vi "Instrument.Lockin.TestLauncher.vi"() -> ()   [LabVIEW 2019, in "Instrument.Lockin.lvlib" / "Instrument.Lockin.lvclass"]
uses:
  Instrument.Lockin.lvclass
  Instrument UI.Lockin/Instrument UI.Lockin.lvclass
  <userlib>/LevyLab/Instrument Framework/Instrument UI/Instrument UI.lvclass
  <userlib>/LevyLab/Instrument Framework/Instrument/Instrument.lvclass
  C:/Program Files (x86)/National Instruments/LabVIEW 2019/user.lib/LevyLab/Instrument Framework/Instrument Types/Lockin/Instrument.LockinAPI.lvclass
  C:/Program Files (x86)/National Instruments/LabVIEW 2019/user.lib/LevyLab/Instrument Framework/Instrument/Instrument.lvclass
  C:/Program Files (x86)/National Instruments/LabVIEW 2019/vi.lib/JKI/JKI SMO/SMO/SMO.lvclass
  <vilib>/JKI/JKI SMO/SMO/SMO.lvclass
  <vilib>/JKI/JKI SMO/SMO.UI/SMO.UI.lvclass
  <vilib>/JKI/JKI SMO/SMO/Typedefs/SMOState --Enum.ctl
  C:/Program Files (x86)/National Instruments/LabVIEW 2019/user.lib/LevyLab/Instrument Framework/Instrument UI/Instrument UI.lvclass
  C:/Program Files (x86)/National Instruments/LabVIEW 2019/vi.lib/JKI/JKI SMO/SMO.UI/SMO.UI.lvclass
  <vilib>/JKI/JKI SMO/SMO/Typedefs/Reserve State--Enum.ctl
  <vilib>/JKI/JKI SMO/SMO/Typedefs/Public Events.ctl
panel:
  out "String":string
  in  "Debug Mode? [F]":bool
  out "UI SMO State":T1
  out "SMO State":T1
  out "error out":errorcluster
  in  "Stop":bool
  # "Example Instrument SMO Test Launcher"
  # "For instructions on how to use the JKI State Machine Objects, examples and video tutorials, visit:\nhttp://jki.net/state-machine-objects/\n\nJKI State Machine Objects™\nhttp://jki.net/state-machine-objects/\nCopyright (C) 2005-2015, JKI <info@jki.net>\nALL RIGHTS RESERVED"
  # "Starting Example Instrument..."
  # "Close Panel to stop the SMO\n(press the \"X\")"
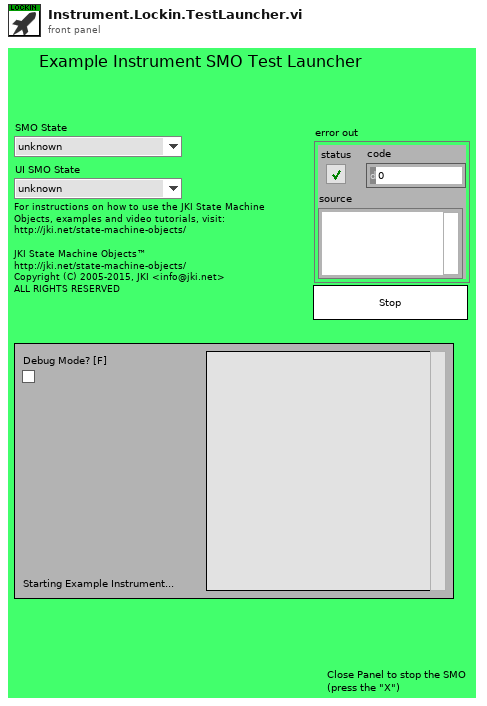
[diagram p1: front panel]
types:
  T1 = typedef "SMO.lvclass/SMOState --Enum.ctl" = enum16{"unknown", "Created", "Started", "Stopped"}
  T2 = typedef "SMO.lvclass/Public Events.ctl" = cluster{"Error":refnum<user-event>, "State":refnum<user-event>, "Reserve State":refnum<user-event>}
  T3 = enum32{"Invalid", "Standard", "Closed", "Hidden", "Minimized", "Maximized"}
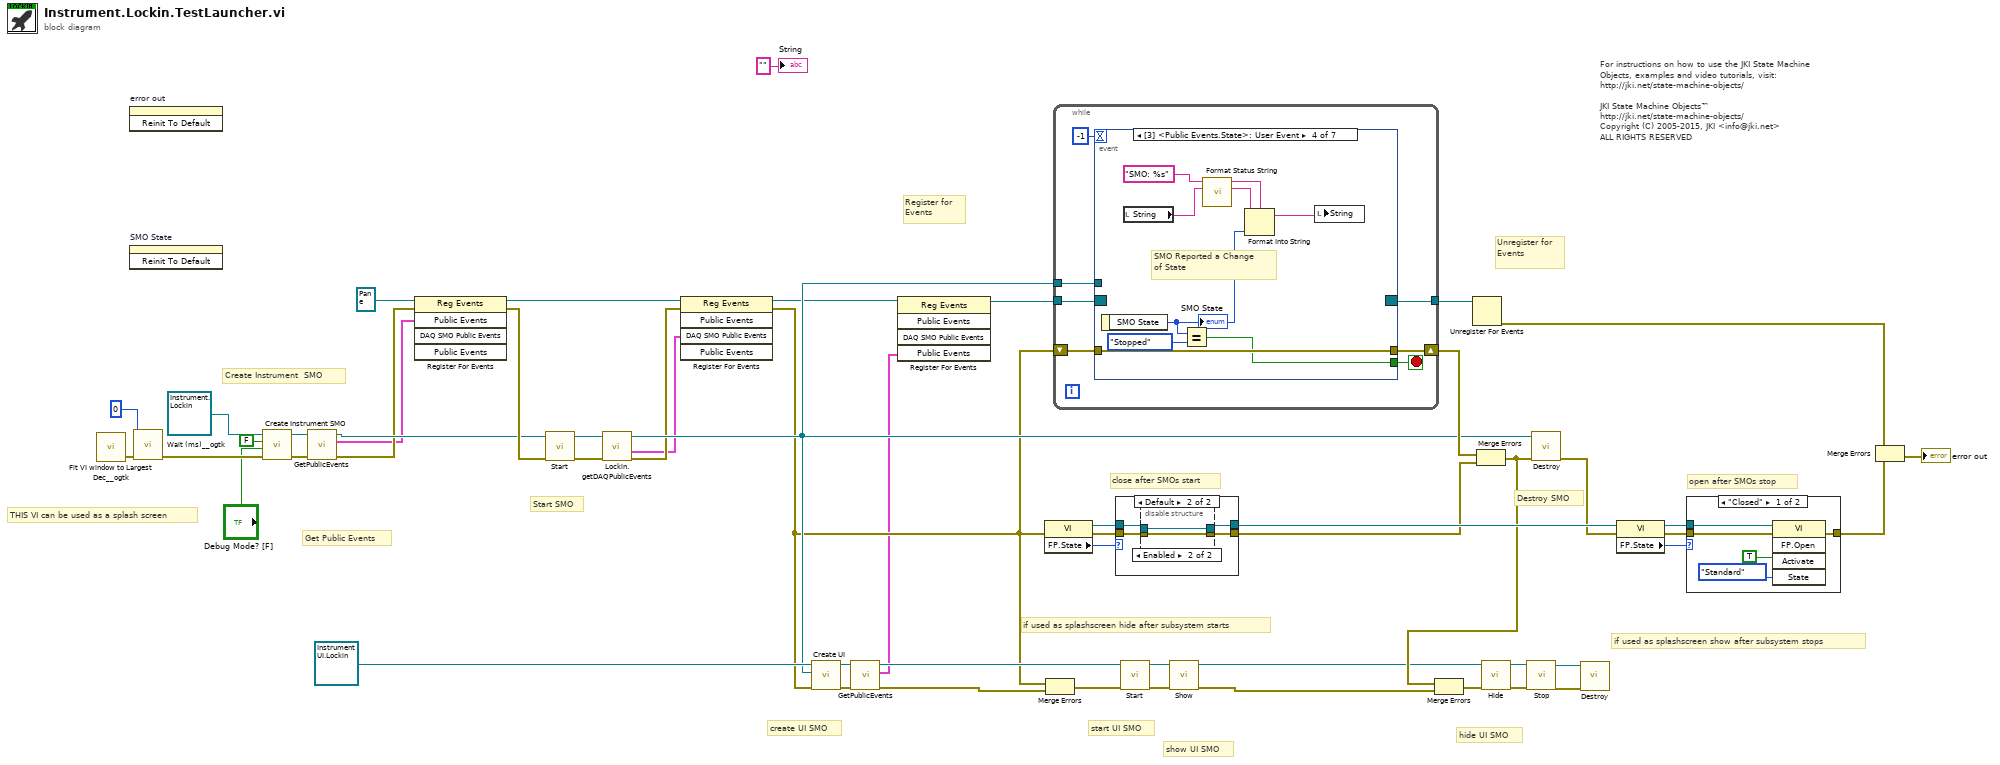
[diagram p0: block diagram]
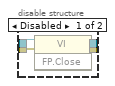
[diagram p3: hidden frame]
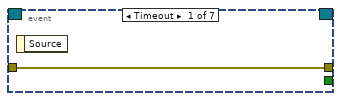
[diagram p5: hidden frame]
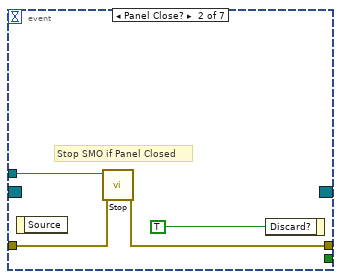
[diagram p6: hidden frame]
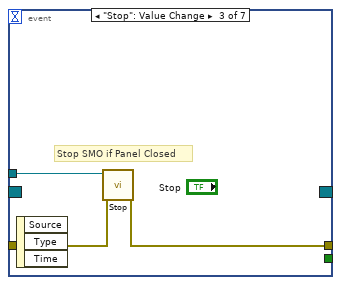
[diagram p7: hidden frame]
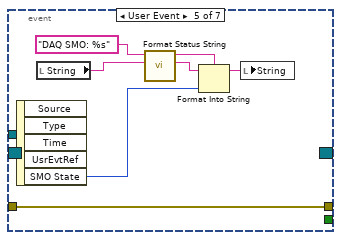
[diagram p8: hidden frame]
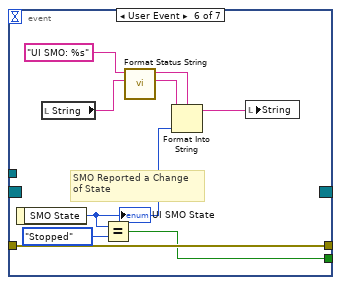
[diagram p9: hidden frame]
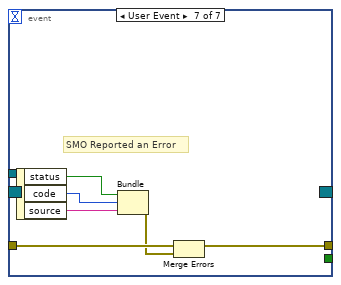
[diagram p10: hidden frame]
diagram:
  # "close after SMOs start"
  # "open after SMOs stop"
  # "hide UI SMO"
  # "show UI SMO"
  # "start UI SMO"
  # "create UI SMO"
  # "if used as splashscreen show after subsystem stops"
  # "if used as splashscreen hide after subsystem starts"
  # "THIS VI can be used as a splash screen"
  # "Get Public Events"
  # "Start SMO"
  # "Destroy SMO"
  # "Create Instrument  SMO"
  # "Unregister for Events"
  # "Register for Events"
  # "For instructions on how to use the JKI State Machine Objects, examples and video tutorials, visit:\nhttp://jki.net/state-machine-objects/\n\nJKI State Machine Objects™\nhttp://jki.net/state-machine-objects/\nCopyright (C) 2005-2015, JKI <info@jki.net>\nALL RIGHTS RESERVED"
  n1 = call <userlib>:"Fit VI window to Largest Dec__ogtk.vi"() -> ("error out"=w43:errorcluster)  [unwired: 6 in, 1 out]
  n2 = invoke on="error out" class="Clust (strict)" method="Reinit To Default"() -> ()  [unwired: 3 in, 3 out]
  n3 = invoke on="SMO State" class="Enum (strict)" method="Reinit To Default"() -> ()  [unwired: 3 in, 3 out]
  n4 = call <userlib>:"Wait (ms)__ogtk.vi"("error in (no error)"=w43, "milliseconds to wait"=u32 0) -> ("error out"=w26:errorcluster)  [unwired: 8 in, 1 out]
  n5 = call <userlib>:"Create Instrument SMO.vi"("error in (no error)"=w26, "Debug Mode? [F]"="Debug Mode? [F]", "Configuration Window? [T]"=FALSE, "Instrument in"=refnum<class "Instrument.Lockin.lvclass"> refnum ("SMO.Template.lvclass")) -> ("error out"=w49:errorcluster, "Instrument out"=w50:refnum<class "Instrument.Lockin.lvclass">)  [unwired: 6 in]
  n6 = call <vilib>:"GetPublicEvents.vi"("error in (no error)"=w49, "SMO"=w50) -> ("error out"=w9:errorcluster, "Public Events"=w4:T2, "SMO out"=w11:refnum<class "Instrument.Lockin.lvclass">)  [unwired: 7 in]
  n7 = register-events(reference=refnum<event-registration> refnum ("event registration refnum"), error in=w9, w4) -> (reference out=w15:refnum<event-registration>, error out=w14:errorcluster)  [unwired: 2 in]
  n8 = call <vilib>:"Start.vi"("error in (no error)"=w14, "SMO"=w11) -> ("error out"=w13:errorcluster, "SMO out"=w12:refnum<class "Instrument.Lockin.lvclass">)  [unwired: 8 in]
  n9 = call "Lockin.getDAQPublicEvents.vi"("error in (no error)"=w13, "Instrument.Lockin in"=w12) -> ("error out"=w7:errorcluster, "DAQ SMO Public Events"=w3:T2, "Instrument.Lockin out"=w10:refnum<class "Instrument.Lockin.lvclass">)  [unwired: 6 in, 1 out]
  n10 = register-events(reference=w15, error in=w7, w3) -> (reference out=w8:refnum<event-registration>, error out=w6:errorcluster)  [unwired: 2 in]
  n11 = call <userlib>:"Create UI.vi"("error in (no error)"=w6, "Instrument in"=w10, "Instrument UI"=refnum<class "Instrument UI.Lockin.lvclass"> refnum ("Lockin.UI")) -> ("error out"=w42:errorcluster, "Instrument UI out"=w41:refnum<class "Instrument UI.Lockin.lvclass">)  [unwired: 7 in]
  n12 = call <vilib>:"GetPublicEvents.vi"("error in (no error)"=w42, "SMO"=w41) -> ("error out"=w5:errorcluster, "Public Events"=w2:T2, "SMO out"=w17:refnum<class "Instrument UI.Lockin.lvclass">)  [unwired: 7 in]
  n13 = register-events(reference=w8, w2) -> (reference out=w16:refnum<event-registration>)  [unwired: 3 in, 1 out]
  n14 = property class="VI"(error in=w6) -> (reference out=w20:refnum<vi>, error out=w21:errorcluster, "FP.State"=w19:T3)  [unwired: 1 in]
  n15 = Merge Errors(w6, w5) -> (w40:errorcluster)
  n16 = while {
    shift-right: [w60] -> w48
    shift-left: w6 -> [w59]
    tunnel: w16 -> [w58]
    tunnel: [w57] -> w53
    tunnel: w10 -> [w56]
    stop <- w61 stop-if-true
    n17 = event shown="[3] <Public Events.State>: User Event" {
      selector: w58 -> [_ _ _ _ _ _ _]
      dyn-events: [_ _ _ _ _ _ _] -> w57
      timeout: -1 -> [_ _ _ _ _ _ _]
      tunnel: [_ _ _ w76 _ w92 _] -> w61
      tunnel: w56 -> [_ w66 w69 _ _ _ _]
      tunnel: [w62 w65 w68 w78 w83 w94 w98] -> w60
      tunnel: w59 -> [w62 w64 w67 w78 w83 w94 w96]
      event Timeout {
        n18 = event-data() -> ()  [unwired: 1 in, 1 out]
      }
      event Panel Close? {
        # "Stop SMO if Panel Closed"
        n19 = event-data() -> ()  [unwired: 1 in, 1 out]
        n20 = call <vilib>:"Stop.vi"("error in (no error)"=w64, "SMO"=w66) -> ("error out"=w65:errorcluster)  [unwired: 8 in, 1 out]
        n21 = event-data("Discard?"=TRUE ("OK")) -> ()  [unwired: 1 in, 1 out]
      }
      event "Stop": Value Change {
        # "Stop SMO if Panel Closed"
        n22 = event-data() -> ()  [unwired: 1 in, 3 out]
        n23 = call <vilib>:"Stop.vi"("error in (no error)"=w67, "SMO"=w69) -> ("error out"=w68:errorcluster)  [unwired: 8 in, 1 out]
      }
      event User Event {
        # "SMO Reported a Change\nof State"
        n24 = event-data() -> ("SMO State"=w74:T1)  [unwired: 1 in]
        "SMO State" <- w74
        n25 = local read "String"() -> (w72:string)
        n26 = Equal?(x=w74, y=SMOState_--Enum."Stopped") -> (x = y?=w76:bool)
        n27 = call "Format Status String.vi"("initial string"=w72, "format string"="SMO: %s") -> ("initial string out"=w71:string, "format string out"=w70:string)  [unwired: 8 in]
        n28 = Format Into String(format string=w70, initial string=w71, w74) -> (resulting string=w75:string)  [unwired: 1 in, 1 out]
        n29 = local write "String"(w75) -> ()
      }
      event User Event {
        n30 = event-data() -> ("SMO State"=w85:T1)  [unwired: 1 in, 4 out]
        n31 = local read "String"() -> (w82:string)
        n32 = call "Format Status String.vi"("initial string"=w82, "format string"="DAQ SMO: %s") -> ("initial string out"=w79:string, "format string out"=w80:string)  [unwired: 8 in]
        n33 = Format Into String(format string=w80, initial string=w79, w85) -> (resulting string=w84:string)  [unwired: 1 in, 1 out]
        n34 = local write "String"(w84) -> ()
      }
      event User Event {
        # "SMO Reported a Change\nof State"
        n35 = event-data() -> ("SMO State"=w90:T1)  [unwired: 1 in]
        "UI SMO State" <- w90
        n36 = local read "String"() -> (w89:string)
        n37 = Equal?(x=w90, y=SMOState_--Enum."Stopped") -> (x = y?=w92:bool)
        n38 = call "Format Status String.vi"("initial string"=w89, "format string"="UI SMO: %s") -> ("initial string out"=w87:string, "format string out"=w86:string)  [unwired: 8 in]
        n39 = Format Into String(format string=w86, initial string=w87, w90) -> (resulting string=w91:string)  [unwired: 1 in, 1 out]
        n40 = local write "String"(w91) -> ()
      }
      event User Event {
        # "SMO Reported an Error"
        n41 = event-data() -> ("status"=w97:bool, "code"=w100:i32, "source"=w99:string)  [unwired: 1 in]
        n42 = Bundle("status"=w97, "code"=w100, "source"=w99) -> (w95:errorcluster)  [unwired: 1 in]
        n43 = Merge Errors(w96, w95) -> (w98:errorcluster)
      }
    }
  }
  n44 = case shown="Default" w19 {
    tunnel: [w102 w106] -> w44
    tunnel: w21 -> [w102 w105]
    tunnel: w20 -> [w101 w104]
    tunnel: [w101 w103] -> w47
    frame "Invalid", "Closed" {
    }
    frame Default {
      n45 = disable-structure shown="Enabled" {
        disable-tunnel: [w110 w111] -> w106
        disable-tunnel: w105 -> [w109 w111]
        disable-tunnel: w104 -> [w108 w112]
        disable-tunnel: [w107 w112] -> w103
        frame Disabled {
          n46 = invoke class="VI" method="FP.Close"(reference=w108, error in=w109) -> (reference out=w107:refnum<vi>, error out=w110:errorcluster)  [unwired: 1 in, 1 out]
        }
        frame Enabled {
        }
      }
    }
  }
  n47 = call <vilib>:"Start.vi"("error in (no error)"=w40, "SMO"=w17) -> ("error out"=w36:errorcluster, "SMO out"=w35:refnum<class "Instrument UI.Lockin.lvclass">)  [unwired: 8 in]
  n48 = call <vilib>:"Show.vi"("error in (no error)"=w36, "SMO.UI"=w35) -> ("error out"=w34:errorcluster, "SMO.UI out"=w30:refnum<class "Instrument UI.Lockin.lvclass">)  [unwired: 8 in]
  n49 = Unregister For Events(event registration refnum=w53) -> (error out=w52:errorcluster)  [unwired: 1 in]
  n50 = Merge Errors(w48, w44) -> (w37:errorcluster)
  n51 = Merge Errors(w37, w34) -> (w31:errorcluster)
  n52 = call <vilib>:"Hide.vi"("error in (no error)"=w31, "SMO.UI"=w30) -> ("error out"=w33:errorcluster, "SMO.UI out"=w32:refnum<class "Instrument UI.Lockin.lvclass">)  [unwired: 8 in]
  n53 = call <vilib>:"Stop.vi"("error in (no error)"=w33, "SMO"=w32) -> ("error out"=w39:errorcluster, "SMO out"=w38:refnum<class "Instrument UI.Lockin.lvclass">)  [unwired: 8 in]
  n54 = call <vilib>:"Destroy.vi"("error in (no error)"=w37, "SMO"=w10) -> ("error out"=w46:errorcluster)  [unwired: 9 in]
  n55 = call <vilib>:"Destroy.vi"("error in (no error)"=w39, "SMO"=w38) -> ()  [unwired: 9 in, 1 out]
  n56 = property class="VI"(reference=w47, error in=w46) -> (reference out=w28:refnum<vi>, error out=w29:errorcluster, "FP.State"=w27:T3)
  n57 = case shown="\"Closed\"" w27 {
    tunnel: [w115 w118] -> w45
    tunnel: w29 -> [w114 w118]
    tunnel: w28 -> [w113 _]
    frame "Closed" {
      n58 = invoke class="VI" method="FP.Open"(reference=w113, error in=w114, "Activate"=TRUE, "State"=T3."Standard") -> (error out=w115:errorcluster)  [unwired: 1 in, 4 out]
    }
    frame Default {
    }
  }
  n59 = Merge Errors(w52, w45) -> (→"error out":errorcluster)
  "String" <- "" ("String")
